vi "SwissSPAD Live_Settings Event Refnum.vi"(1 "Settings Event":T1, 3 "Error In":errorcluster) -> (7 "Settings Event Refnum":refnum<user-event>, 9 "Error Out":errorcluster)   [LabVIEW 2021]
uses:
  SwissSPAD Live_Settings Event.ctl
  SwissSPAD Live_Settings Window Messages.ctl
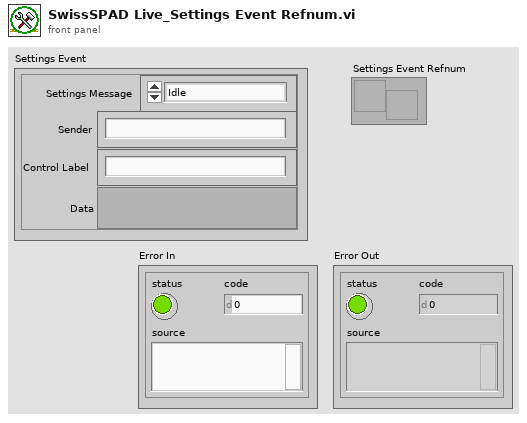
[diagram p1: front panel]
types:
  T1 = typedef "SwissSPAD Live_Settings Event.ctl" = cluster{"Settings Message":T2, "Sender":string, "Control Label":string, "Data":variant}
  T2 = typedef "SwissSPAD Live_Settings Window Messages.ctl" = enum16{"Idle", "Subscribe", "Unsubscribe", "Refresh Parameter", "Refresh All Parameters", "Quit"}
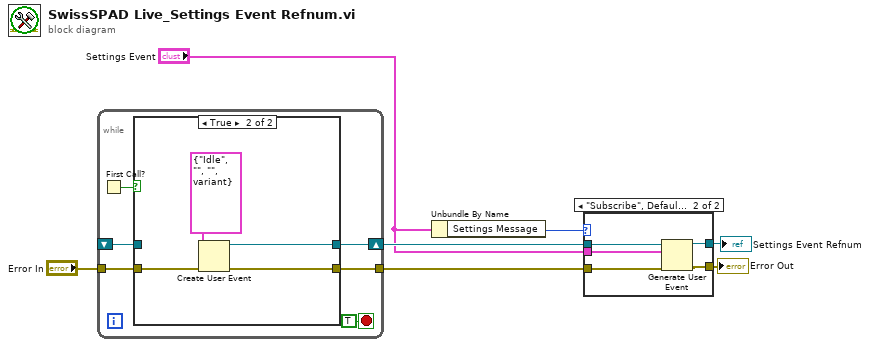
[diagram p0: block diagram]
diagram:
  n1 = while {
    shift-right: [w11] -> w5
    shift-left: _ -> [w10]
    tunnel: [w9] -> w6
    tunnel: "Error In" -> [w8]
    stop <- TRUE stop-if-true
    n2 = First Call?() -> (First Call?: T/F=w13:bool)
    n3 = case shown="True" w13 {
      tunnel: [w15 w19] -> w11
      tunnel: w10 -> [w15 _]
      tunnel: [w14 w18] -> w9
      tunnel: w8 -> [w14 w17]
      frame False {
      }
      frame True {
        n4 = Create User Event(user event datatype=T1 {"Settings Message"=enum."Idle", "Sender"="", "Control Label"="", "Data"=variant} ("Settings Event"), error in=w17) -> (user event=w19:refnum<user-event>, error out=w18:errorcluster)
      }
    }
  }
  n5 = Unbundle By Name("Settings Event") -> ("Settings Message"=w2:T2)
  n6 = case shown="\"Subscribe\", Default" w2 {
    tunnel: w6 -> [w20 w26]
    tunnel: w5 -> [w21 w25]
    tunnel: [w20 w24] -> w4
    tunnel: "Settings Event" -> [_ w23]
    tunnel: [w21 w22] -> w1
    frame "Idle" {
    }
    frame "Subscribe", Default {
      n7 = Generate User Event(user event=w25, event data cluster=w23, error in=w26) -> (user event out=w22:refnum<user-event>, error out=w24:errorcluster)  [unwired: 1 in]
    }
  }
  "Error Out" <- w4
  "Settings Event Refnum" <- w1
